vi "Disconnect.vi"(0 "MB_MODULE":refnum<class "MB_MODULE.lvclass">, 11 "error in":errorcluster) -> (15 "error out":errorcluster)   [LabVIEW 2019, in "MB_MODULE.lvclass"]
uses:
  MB_MODULE.lvclass
  MB_MODULE.lvclass/MB_MODULE.ctl
  <vilib>/NI/Modbus Library/API/Master/Modbus Master.lvclass
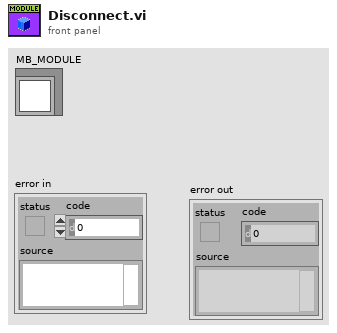
[diagram p1: front panel]
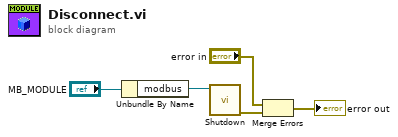
[diagram p0: block diagram]
diagram:
  n1 = Unbundle By Name("MB_MODULE") -> ("modbus"=w4:refnum<class "Modbus Master.lvclass">)
  n2 = call-dynamic "Shutdown.vi"("Modbus master in"=w4) -> ("error out"=w3:errorcluster)  [unwired: 10 in]
  n3 = Merge Errors("error in", w3) -> (→"error out":errorcluster)
